vi "CF_Z_Bridge_to_DSC.vi"(0 "description, string":refnum<k21>="ni.var.psp://housesoftheholy/Leiden CF900/CF_TC_Z_description", 1 "dbl var":refnum<k21>[](array[refnum])=["ni.var.psp://housesoftheholy/Leiden CF900/CF_TC_Z_R0", "ni.var.psp://housesoftheholy/Leiden CF900/CF_TC_Z_R1", "ni.var.psp://housesoftheholy/Leiden CF900/CF_TC_Z_R2", "ni.var.psp://housesoftheholy/Leiden CF900/CF_TC_Z_R3", "ni.var.psp://housesoftheholy/Leiden CF900/CF_TC_Z_R4", "ni.var.psp://housesoftheholy/Leiden CF900/CF_TC_Z_R5", "ni.var.psp://housesoftheholy/Leiden CF900/CF_TC_Z_R6", "ni.var.psp://housesoftheholy/Leiden CF900/CF_TC_Z_R7", "ni.var.psp://housesoftheholy/Leiden CF900/CF_TC_Z_R8", "ni.var.psp://housesoftheholy/Leiden CF900/CF_TC_Z_R9", "ni.var.psp://housesoftheholy/Leiden CF900/CF_TC_Z_T0", "ni.var.psp://housesoftheholy/Leiden CF900/CF_TC_Z_T1", "ni.var.psp://housesoftheholy/Leiden CF900/CF_TC_Z_T2", "ni.var.psp://housesoftheholy/Leiden CF900/CF_TC_Z_T3", "ni.var.psp://housesoftheholy/Leiden CF900/CF_TC_Z_T4", "ni.var.psp://housesoftheholy/Leiden CF900/CF_TC_Z_T5", "ni.var.psp://housesoftheholy/Leiden CF900/CF_TC_Z_T6", "ni.var.psp://housesoftheholy/Leiden CF900/CF_TC_Z_T7", "ni.var.psp://housesoftheholy/Leiden CF900/CF_TC_Z_T8", "ni.var.psp://housesoftheholy/Leiden CF900/CF_TC_Z_T9"], 2 "dbl":dbl[](array[numeric])=[-1e+30, 3977.4776241280374, 3649.809852131724, 0.0, 17313.58847758918, 0.0, 0.0, 0.0, 0.0, 0.0, -5.724e-36, 4025.436136585684, 4054.3239935153424, nan, 4258.3107502810735, 0.0, 0.0, 0.0, 0.0, 0.0], 5 "String In":string="3K, Still, 50 mK, MC, MC, , , , , ", 7 "calibration string":refnum<k21>="ni.var.psp://housesoftheholy/Leiden CF900/CF_TC_Z_calibration", 9 "String In 2":string="CMN 187_TC_2-29, 140701_OuterSP (fit from fit, self defined fx)_TC, 140702_Solenoid (Right, fit from fit, self defined fx)_TC, RuO2_10K_TC, RuO2_10K_TC, No Calibration, No Calibration, No Calibration, No Calibration, No Calibration") -> ()   [LabVIEW 2013]
panel:
  # "CF Impedence Bridge to DSC"
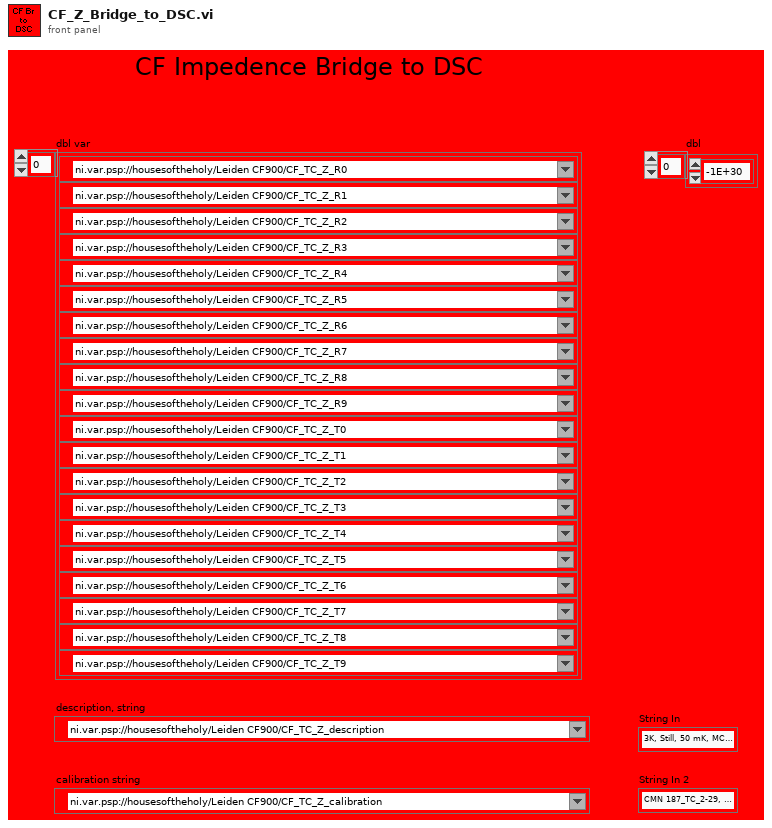
[diagram p1: front panel]
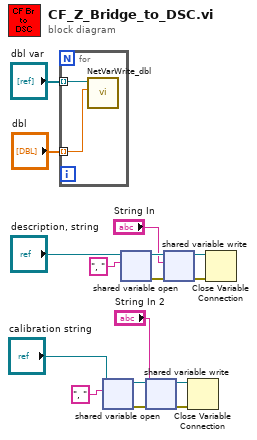
[diagram p0: block diagram]
diagram:
  n1 = for {
    tunnel: "dbl var" -> [w18] mode=indexing
    tunnel: "dbl" -> [w17] mode=indexing
    n2 = call "NetVarWrite_dbl.vi"("Numeric"=w17, "Refnum in"=w18) -> ()  [unwired: 10 in]
  }
  n3 = shared-variable-open("calibration string", ", " ("string")) -> (w6:refnum<k21>, w5:errorcluster)  [unwired: 2 in]
  n4 = shared-variable-open("description, string", ", " ("string")) -> (w13:refnum<k21>, w12:errorcluster)  [unwired: 2 in]
  n5 = shared-variable-write(w6, w5, "String In 2") -> (w7:refnum<k21>, w4:errorcluster)
  n6 = shared-variable-write(w13, w12, "String In") -> (w14:refnum<k21>, w11:errorcluster)
  n7 = Close Variable Connection(8:w4, 11:w7) -> ()  [unwired: 1 out]
  n8 = Close Variable Connection(8:w11, 11:w14) -> ()  [unwired: 1 out]
